vi "KE24xx, Setup.vi"(5 "Active Terminals (Rear)":u16(ring)=1 items=["Front", "Rear"], 6 "error in":errorcluster, 7 "Reset (True)":bool=TRUE, 8 "ID Query (True)":bool=TRUE, 9 "VISA rsrc":refnum<visa-resource-name>) -> (0 "error out":errorcluster, 3 "VISA rsrc out":refnum<visa-resource-name>)   [LabVIEW 2010]
doc: "This function establishes communication with the SMU and optionally performs an instrument identification query and/or an instrument reset. It also places the instrument in a default state needed for other instrument driver operations. \n\nGenerally, you need to call this function only once at the beginning of an application."
uses:
  <instrlib>/Keithley 24XX/Keithley 24XX.lvlib
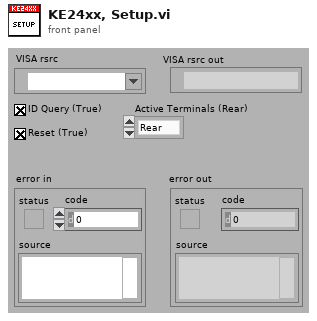
[diagram p1: front panel]
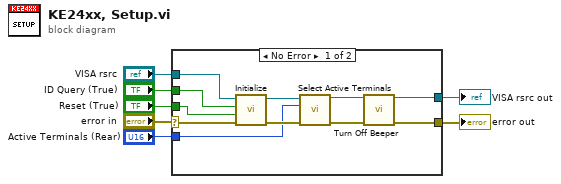
[diagram p0: block diagram]
diagram:
  n1 = case shown="No Error" "error in" {
    selector: "error in" -> [w18 w20]
    tunnel: [w11 w20] -> w6
    tunnel: "Reset (True)" -> [w17 _]
    tunnel: "ID Query (True)" -> [w16 _]
    tunnel: "VISA rsrc" -> [w15 w19]
    tunnel: "Active Terminals (Rear)" -> [w13 _]
    tunnel: [w8 w19] -> w1
    frame No Error {
      n2 = call <instrlib>:"Initialize.vi"("error in (no error)"=w18, "Reset (True)"=w17, "ID Query (True)"=w16, "VISA resource name"=w15) -> ("error out"=w14:errorcluster, "VISA resource name out"=w9:refnum<visa-resource-name>)  [unwired: 6 in]
      n3 = call <instrlib>:"Select Active Terminals.vi"("error in (no error)"=w14, "Active Terminals (0: Front)"=w13, "VISA resource name"=w9) -> ("error out"=w12:errorcluster, "VISA resource name out"=w10:refnum<visa-resource-name>)  [unwired: 7 in]
      n4 = call "Turn Off Beeper.vi"("VISA resource name"=w10, "error in (no error)"=w12) -> ("VISA resource name out"=w8:refnum<visa-resource-name>, "error out"=w11:errorcluster)  [unwired: 12 in]
    }
    frame Error {
    }
  }
  "VISA rsrc out" <- w1
  "error out" <- w6
